vi "set date.vi"(8 "error in (no error)":errorcluster caption="Fehler (Eingang, kein Fehler)", 10 "date":string, 11 "Report (Eingang)":refnum<class "Report.lvclass">) -> (0 "error out":errorcluster caption="Fehler (Ausgang)", 3 "Report (Ausgang)":refnum<class "Report.lvclass">)   [LabVIEW 2013, in "DatenKlassen.lvlib" / "Report.lvclass"]
uses:
  Report.lvclass
  Report.lvclass/Report.ctl
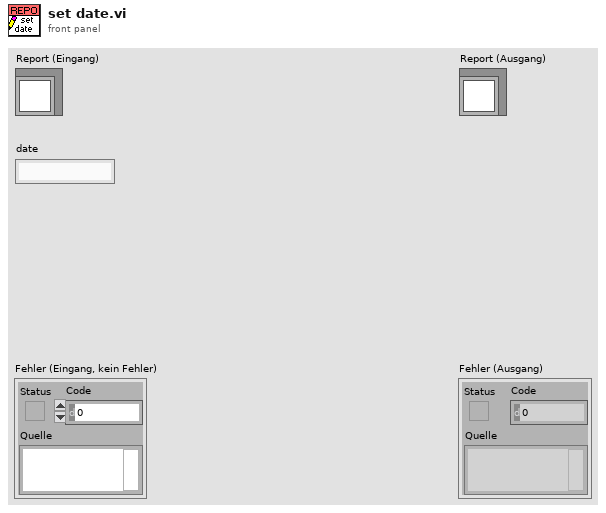
[diagram p1: front panel]
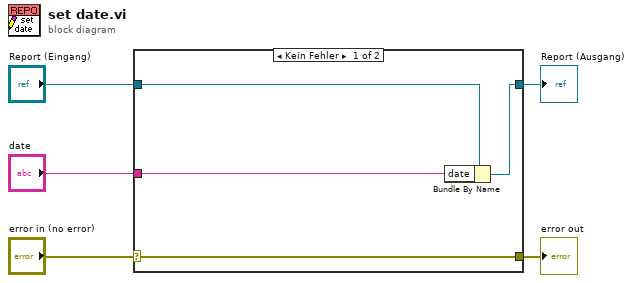
[diagram p0: block diagram]
diagram:
  n1 = case shown="Kein Fehler" "error in (no error)" {
    selector: "error in (no error)" -> [w9 w10]
    tunnel: [w9 w10] -> w4
    tunnel: [w7 w11] -> w2
    tunnel: "Report (Eingang)" -> [w8 w11]
    tunnel: "date" -> [w6 _]
    frame No Error {
      n2 = Bundle By Name(cluster=w8, "date"=w6) -> (w7:refnum<class "Report.lvclass">)
    }
    frame Error {
    }
  }
  "error out" <- w4
  "Report (Ausgang)" <- w2
